vi "4.6.1.vi"() -> ()   [LabVIEW 2018]
panel:
  out "배열 4":i32[][](array[numeric])
  out "배열 3":i32[](array[numeric])
  out "배열 2":i32[](array[numeric])
  out "숫자형":i32
  out "배열":i32[](array[numeric])
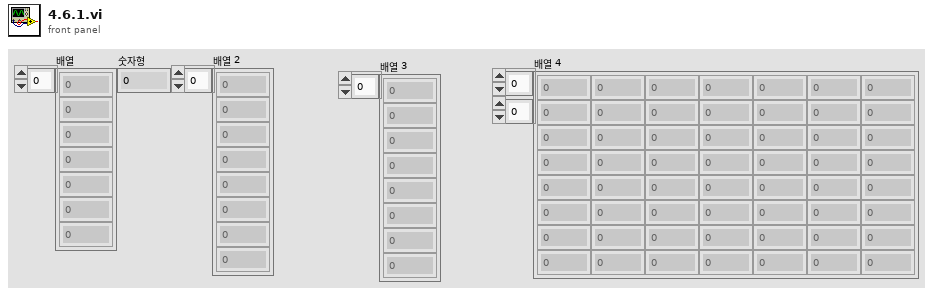
[diagram p1: front panel]
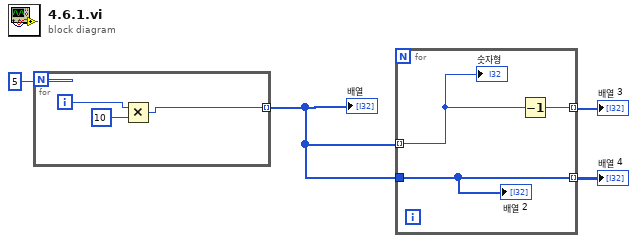
[diagram p0: block diagram]
diagram:
  n1 = for {
    N: 5 -> [_]
    tunnel: [w5] -> w3 mode=indexing
    i -> [w7]
    n2 = Multiply(x=w7, y=10) -> (x*y=w5:i32)
  }
  "배열" <- w3
  n3 = for {
    tunnel: w3 -> [w10] mode=indexing
    tunnel: w3 -> [w8]
    tunnel: [w9] -> w2 mode=indexing
    tunnel: [w8] -> w1 mode=indexing
    n4 = Decrement(x=w10) -> (x-1=w9:i32)
    "숫자형" <- w10
    "배열 2" <- w8
  }
  "배열 3" <- w2
  "배열 4" <- w1
